vi "Framework Source Test.vi"() -> ()   [LabVIEW 2017]
uses:
  Typedefs/DSF Engine Framework Configuration.ctl
  Typedefs/DSF Engine Plugin Configuration.ctl
  Typedefs/DSF Timing Info.ctl
  Typedefs/DSF Engine Plugin Thread Configuration.ctl
  Typedefs/DSF Settings Info.ctl
  Typedefs/DSF Engine Transfer Group Configuration.ctl
  Typedefs/DSF Direction.ctl
  Typedefs/DSF Engine Transfer Configuration.ctl
  Typedefs/DSF Byte Order.ctl
  Typedefs/DSF Engine Channel Configuration.ctl
  Typedefs/DSF Data Type.ctl
  Typedefs/DSF Timeout Behavior.ctl
  Classes/Framework/Framework Options.ctl
  Typedefs/DSF FIFO Options.ctl
  Classes/Thread/DSF Thread Options.ctl
  Typedefs/DSF Plugin Options.ctl
  Typedefs/DSF Performance Options.ctl
  <vilib>/NI/Memory Manager/Classes/Pointer/Pointer.lvclass/Pointer.ctl
  Classes/Framework/Framework.lvclass/Framework.ctl
  Classes/Performance/Performance.lvclass/Performance.ctl
  Classes/Plugin/Plugin.lvclass/Plugin.ctl
  Classes/Timing/Timing.lvclass/Timing.ctl
  Classes/Transfer Group/Transfer Group.lvclass/Transfer Group.ctl
  Classes/Interface/Interface.lvclass/Interface.ctl
  Classes/Buffers/Buffers.lvclass/Buffers.ctl
  Classes/Framework Status/Framework Status.lvclass/Framework Status.ctl
  <vilib>/NI/Memory Manager/Classes/Pointer/Write Bool.vi
  <vilib>/NI/Memory Manager/Classes/Pointer/Set Address.vi
  <vilib>/NI/Memory Manager/Classes/Pointer/Set Size.vi
  <vilib>/NI/Memory Manager/Classes/Pointer/Set Internal.vi
  <vilib>/NI/Memory Manager/Classes/Pointer/Write (No Check).vi
  <vilib>/NI/Memory Manager/Classes/Pointer/Write (No Check) Bool.vi
  <vilib>/NI/Memory Manager/Classes/Pointer/Check Move.vi
  <vilib>/NI/Memory Manager/Classes/Pointer/Check Null Pointer.vi
  <vilib>/NI/Memory Manager/Classes/Pointer/Clear (No Check).vi
  <vilib>/NI/Memory Manager/Classes/Pointer/Check Length.vi
  <vilib>/NI/Memory Manager/Classes/Pointer/Read (No Check).vi
  <vilib>/NI/Memory Manager/Classes/Pointer/Read (No Check) Bool.vi
  Classes/Framework/Active Plugins.vi
  Classes/Framework/Rx Begin.vi
  Classes/Framework/Rx End.vi
  Classes/Framework/Rx Inline Wait.vi
  Classes/Framework/Rx Async.vi
  Classes/Framework/Rx Inline Start.vi
  Classes/Framework/No Inline Plugins.vi
  Classes/Framework/No Async Plugins.vi
  Classes/Framework/Tx End.vi
  Classes/Framework/Tx Begin.vi
  Classes/Framework/Tx Inline Start.vi
  Classes/Framework/Tx Async.vi
  Classes/Framework/Tx Inline Wait.vi
  Classes/Framework/Update Performance.vi
  Classes/Framework/Update Status.vi
  Classes/Framework/Increment Plugins.vi
  <vilib>/NI/Memory Manager/Classes/Pointer/Get Internal.vi
  <vilib>/NI/Memory Manager/Classes/Pointer/Errors.vi
  <vilib>/NI/Memory Manager/Classes/Pointer/Zone.vi
  <vilib>/NI/Memory Manager/Classes/Pointer/Check Count.vi
  <vilib>/NI/Memory Manager/Classes/Pointer/Check Bounds (Power of 2).vi
  <vilib>/NI/Memory Manager/Classes/Pointer/Null Pointer.vi
  <vilib>/NI/Memory Manager/Classes/Pointer/Is Null.vi
  <vilib>/NI/Memory Manager/Classes/Pointer/Check Bounds (Pointer).vi
  Classes/Plugin/Is Active.vi
  Classes/Plugin/Set Active.vi
  Classes/Plugin/Active Transfer Groups.vi
  Classes/Performance/Rx Begin.vi
  Classes/Performance/Rx End.vi
  Classes/Plugin/Rx Inline Wait.vi
  Classes/Plugin/Rx Async.vi
  Classes/Plugin/Rx Inline Start.vi
  Classes/Performance/Tx End.vi
  Classes/Performance/Tx Begin.vi
  Classes/Plugin/Tx Inline Start.vi
  Classes/Plugin/Tx Async.vi
  Classes/Plugin/Tx Inline Wait.vi
  Classes/Performance/Update Timing.vi
  Classes/Status/Write Status.vi
  Classes/Framework Status/Get Framework Pointer.vi
  Classes/Plugin/Update Status.vi
  Classes/Plugin/Increment Iteration.vi
  <vilib>/NI/Memory Manager/Classes/Pointer/Create Error.vi
  <vilib>/NI/Memory Manager/Classes/Pointer/Out of Bounds.vi
  <vilib>/NI/Memory Manager/Classes/Pointer/Check Bounds.vi
  Classes/Timing/Is Active Cycle.vi
  Classes/Transfer Group/Is Active.vi
  Classes/Transfer Group/Set Active.vi
  Classes/Plugin/Iteration.vi
  Classes/Transfer Group/Wait For Previous.vi
  Classes/Transfer Group/Update Status.vi
  Classes/Transfer Group/Increment Iteration.vi
  Classes/Transfer Group/Get Iteration.vi
  Classes/Thread/Dispatcher/Dispatch Transfer Group.vi
  Classes/Transfer Group/Get ID.vi
  Classes/Transfer Group/Copy Async to Inline.vi
  Classes/Transfer Group/Get Active.vi
  Classes/Plugin/Get ID.vi
  Classes/Transfer Group/Copy Inline to Async.vi
  Classes/Performance/Write Timing Status.vi
  Classes/Status/Status Size.vi
  <vilib>/NI/Memory Manager/Classes/Pointer/Check Size.vi
  Classes/Timing/Get Iteration.vi
  Classes/Timing/Increment Iteration.vi
  <vilib>/NI/Memory Manager/Constants/Constants.vi
  <vilib>/NI/Memory Manager/Constants/Library Name.vi
  <vilib>/NI/Memory Manager/Classes/Pointer/Pointer Error Info.vi
  <vilib>/NI/Memory Manager/Constants/Pointer Class Name.vi
  <vilib>/NI/Memory Manager/Classes/Pointer/Write Pointer Size to Error.vi
  <vilib>/NI/Memory Manager/Classes/Pointer/Check Bounds (Buffer).vi
  Classes/Timing/Get Decimation.vi
  Classes/Timing/Get Offset.vi
  Classes/Plugin/Get Timing.vi
  Classes/Transfer Group/Retrieve from FIFO.vi
  Classes/Interface/Dispatcher/Send Dispatcher Command.vi
  Classes/Buffers/Copy Async to Inline.vi
  Classes/Buffers/Copy Inline to Async.vi
  Classes/Timing Status/Write Timing Status.vi
  <vilib>/NI/Memory Manager/Classes/Pointer/Buffer Underflow.vi
  Classes/Transfer Group/Read Return FIFO.vi
  Classes/Transfer Group/Increment Late Count.vi
  Classes/Interface/Dispatcher/Write Dispatcher Command.vi
  <vilib>/NI/Memory Manager/Classes/Pointer/Copy All.vi
  Classes/Timing Status/Timing Status Size.vi
  Classes/Interface/Send Command.vi
  <vilib>/NI/Memory Manager/Classes/Pointer/Copy.vi
  Classes/Interface/Write RT FIFO.vi
  <vilib>/NI/Memory Manager/Classes/Pointer/Copy (No Check).vi
  Classes/Interface/Dispatcher/Dispatcher Interface.lvclass
  C:/Git/DSF/Core/Classes/Interface/Interface.lvclass
  Classes/Buffer/Buffer.lvclass
  C:/Program Files (x86)/National Instruments/LabVIEW 2017/vi.lib/NI/Memory Manager/Classes/Pointer/Pointer.lvclass
  Classes/Status/Status.lvclass
  Classes/Timing Status/Timing Status.lvclass
  <vilib>/NI/Memory Manager/VIs/New Error Cluster.vi
  <vilib>/NI/Memory Manager/VIs/New Error Cluster (512B).vi
  <vilib>/NI/Memory Manager/VIs/Set Error Status.vi
  <vilib>/NI/Memory Manager/VIs/Set Error Code.vi
  <vilib>/NI/Memory Manager/VIs/Set Error Source.vi
  <vilib>/NI/Memory Manager/VIs/Write String to Source.vi
  <vilib>/NI/Memory Manager/VIs/Write Numeric to Source.vi
  <vilib>/NI/Memory Manager/VIs/Write Numeric Scalar to Source (Base10 U64).vi
  Classes/Interface/Dispatcher/Class Name.vi
  VIs/VI Name.vi
  Classes/Interface/Errors.vi
  Classes/Interface/Dispatcher/Command Timeout.vi
  Classes/Transfer Group/Errors.vi
  Classes/Transfer Group/Invalid Iteration Error.vi
  Classes/Transfer Group/Return Timeout Error.vi
  <vilib>/NI/Memory Manager/Classes/Pointer/Pointer.lvclass
  Classes/Framework/Framework.lvclass
  <vilib>/NI/Memory Manager/Classes/Pointer/Read Bool.vi
  Classes/Configuration/Configuration Session.lvclass
  DSF Core.lvlib
panel:
  in  "components directory":path
  in  "dsf configuration file path":path=path "C:/Users/Admin/Desktop/test.dsf"
  out "iteration":u64
  out "error out":errorcluster
  in  "framework options":T1={"FIFO Options"={"Infinite Timeouts"=TRUE}, "Thread Options"={"Show FP On Call"=TRUE, "Close FP After Call"=TRUE, "Allow Debugging"=TRUE}, "Plugin Options"={"Default Components"=TRUE}, "Performance Options"={"Measure Period"=TRUE, "Measure Rx/Tx Duration"=TRUE}}
  in  "framework configuration":T6={"Plugins"=[{"name"="UDP", "components"=["UDP"], "cycle timing"={"priority"=100, "decimation"=1, "offset"=0}, "threads"=[{"buffer converter settings"=[], "transceiver settings"=[{"key"="Local Port", "value"="50000"}], "custom settings"=[], "processor"=-2, "priority offset"=0}, {"buffer converter settings"=[], "transceiver settings"=[{"key"="Local Port", "value"="50001"}], "custom settings"=[], "processor"=-2, "priority offset"=0}, {"buffer converter settings"=[], "transceiver settings"=[{"key"="Local Port", "value"="50002"}], "custom settings"=[], "processor"=-2, "priority offset"=0}, {"buffer converter settings"=[], "transceiver settings"=[{"key"="Local Port", "value"="50003"}], "custom settings"=[], "processor"=-2, "priority offset"=0}], "Transfer Groups"=[{"name"="Group0", "direction"=enum."Tx", "cycle timing"={"priority"=100, "decimation"=1, "offset"=0}, "thread index"=0, "settings"=[], "Transfers"=[{"name"="Transfer0", "byte order"=enum."big-endian", "settings"=[{"key"="Destination Port", "value"="60000"}, {"key"="Destination Address", "value"="localhost"}], "channels"=[{"string offset"=0, "string data type"=enum."SGL", "engine data type"=enum."DBL", "name"="Temp", "settings"=[], "units"="V"}, {"string offset"=4, "string data type"=enum."DBL", "engine data type"=enum."DBL", "name"="RPM", "settings"=[], "units"="V"}, {"string offset"=12, "string data type"=enum."Bool", "engine data type"=enum."DBL", "name"="LED", "settings"=[], "units"="V"}, {"string offset"=792, "string data type"=enum."U64", "engine data type"=enum."DBL", "name"="Count", "settings"=[], "units"="V"}]}], "timeout behavior"=enum."Increment Late Count"}], "settings"=[]}]}
  in  "stop":bool
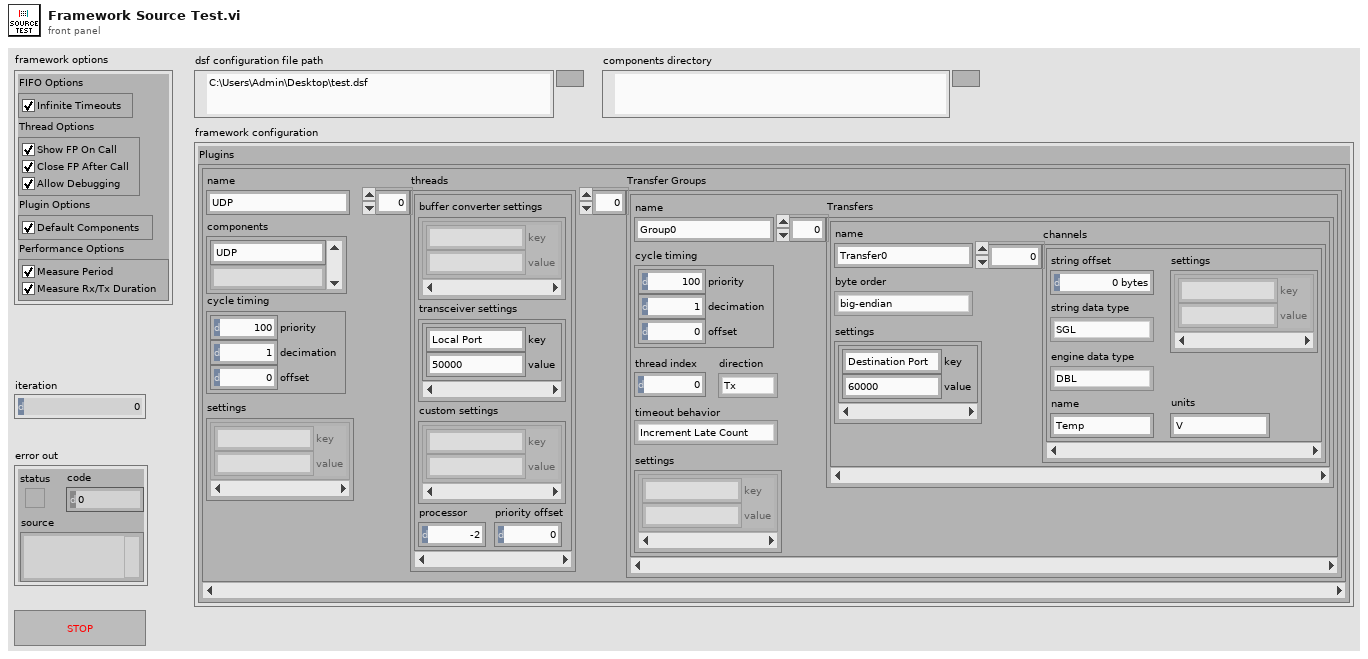
[diagram p1: front panel]
types:
  T1 = typedef "DSF Core.lvlib/Framework.lvclass/Framework Options.ctl" = cluster{"FIFO Options":T2, "Thread Options":T3, "Plugin Options":T4, "Performance Options":T5}
  T2 = typedef "DSF Core.lvlib/DSF FIFO Options.ctl" = cluster{"Infinite Timeouts":bool}
  T3 = typedef "DSF Core.lvlib/DSF Thread Options.ctl" = cluster{"Show FP On Call":bool, "Close FP After Call":bool, "Allow Debugging":bool}
  T4 = typedef "DSF Core.lvlib/DSF Plugin Options.ctl" = cluster{"Default Components":bool}
  T5 = typedef "DSF Core.lvlib/DSF Performance Options.ctl" = cluster{"Measure Period":bool, "Measure Rx/Tx Duration":bool}
  T6 = typedef "DSF Core.lvlib/DSF Engine Framework Configuration.ctl" = cluster{"Plugins":T7[]}
  T7 = typedef "DSF Core.lvlib/DSF Engine Plugin Configuration.ctl" = cluster{"name":string, "components":string[], "cycle timing":T8, "threads":T9[], "Transfer Groups":T11[], "settings":T10}
  T8 = typedef "DSF Core.lvlib/DSF Timing Info.ctl" = cluster{"priority":u64, "decimation":u64, "offset":u64}
  T9 = typedef "DSF Core.lvlib/DSF Engine Plugin Thread Configuration.ctl" = cluster{"buffer converter settings":T10, "transceiver settings":T10, "custom settings":T10, "processor":i32, "priority offset":i16}
  T10 = typedef "DSF Core.lvlib/DSF Settings Info.ctl" = cluster{"key":string, "value":string}[]
  T11 = typedef "DSF Core.lvlib/DSF Engine Transfer Group Configuration.ctl" = cluster{"name":string, "direction":T12, "cycle timing":T8, "thread index":i32, "settings":T10, "Transfers":T13[], "timeout behavior":T17}
  T12 = typedef "DSF Core.lvlib/DSF Direction.ctl" = enum8{"Tx", "Rx"}
  T13 = typedef "DSF Core.lvlib/DSF Engine Transfer Configuration.ctl" = cluster{"name":string, "byte order":T14, "settings":T10, "channels":T15[]}
  T14 = typedef "DSF Core.lvlib/DSF Byte Order.ctl" = enum8{"big-endian", "little-endian"}
  T15 = typedef "DSF Core.lvlib/DSF Engine Channel Configuration.ctl" = cluster{"string offset":u64, "string data type":T16, "engine data type":T16, "name":string, "settings":T10, "units":string}
  T16 = typedef "DSF Core.lvlib/DSF Data Type.ctl" = enum8{"Bool", "SGL", "DBL", "I8", "I16", "I32", "I64", "U8", "U16", "U32", "U64"}
  T17 = typedef "DSF Core.lvlib/DSF Timeout Behavior.ctl" = enum8{"Increment Late Count", "Throw Error"}
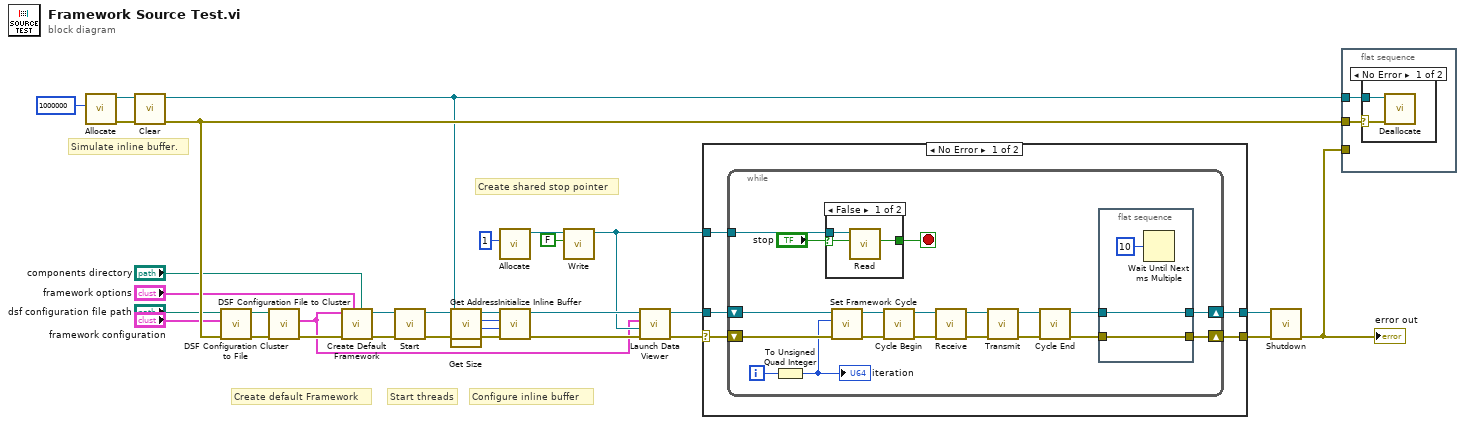
[diagram p0: block diagram]
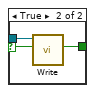
[diagram p3: hidden frame]
diagram:
  # "Create shared stop pointer"
  # "Configure inline buffer"
  # "Start threads"
  # "Create default Framework"
  # "Simulate inline buffer."
  n1 = call <vilib>:"Allocate.vi"("size"=u64 1000000) -> ("error out"=w24:errorcluster, "Pointer out"=w17:refnum<class "Pointer.lvclass">)  [unwired: 9 in]
  n2 = call <vilib>:"Clear.vi"("error in (no error)"=w24, "Pointer in"=w17) -> ("error out"=w29:errorcluster, "Pointer out"=w2:refnum<class "Pointer.lvclass">)  [unwired: 8 in]
  n3 = call "DSF Configuration Cluster to File.vi"("error in (no error)"=w29, "framework configuration"="framework configuration", "dsf configuration file path"="dsf configuration file path") -> ("error out"=w23:errorcluster, "dsf configuration file path dup"=w22:path)  [unwired: 7 in]
  n4 = call "DSF Configuration File to Cluster.vi"("error in (no error)"=w23, "dsf configuration file path"=w22) -> ("error out"=w16:errorcluster, "framework configuration out"=w4:T6)  [unwired: 7 in, 1 out]
  n5 = call "Create Default Framework.vi"("components directory (default)"="components directory", "framework options"="framework options", "error in (no error)"=w16, "framework configuration"=w4) -> ("error out"=w1:errorcluster, "Framework"=w13:refnum<class "Framework.lvclass">)  [unwired: 6 in]
  n6 = call-dynamic "Start.vi"("error in (no error)"=w1, "Framework in"=w13) -> ("error out"=w12:errorcluster, "Framework out"=w30:refnum<class "Framework.lvclass">)  [unwired: 8 in]
  n7 = call <vilib>:"Get Address.vi"("Pointer in"=w2) -> ("address"=w20:u64)  [unwired: 9 in, 1 out]
  n8 = call <vilib>:"Get Size.vi"("Pointer in"=w2) -> ("size"=w21:u64)  [unwired: 9 in, 1 out]
  n9 = call <vilib>:"Allocate.vi"("size"=u64 1) -> ("Pointer out"=w8:refnum<class "Pointer.lvclass">)  [unwired: 9 in, 1 out]
  n10 = call "Initialize Inline Buffer.vi"("error in (no error)"=w12, "size"=w21, "address"=w20, "Framework in"=w30) -> ("error out"=w10:errorcluster, "Framework out"=w11:refnum<class "Framework.lvclass">)  [unwired: 6 in]
  n11 = call-poly <vilib>:"Write.vi"("value"=FALSE, "Pointer in"=w8) -> ("Pointer out"=w7:refnum<class "Pointer.lvclass">)  [unwired: 6 in, 3 out]
  n12 = call "Launch Data Viewer.vi"("error in (no error)"=w10, "Stop Pointer"=w7, "Framework Configuration"=w4, "Framework in"=w11) -> ("error out"=w18:errorcluster, "Framework out"=w19:refnum<class "Framework.lvclass">)  [unwired: 6 in]
  n13 = case shown="No Error" w18 {
    selector: w18 -> [w34 w64]
    tunnel: [w32 w64] -> w28
    tunnel: w19 -> [w35 w65]
    tunnel: [w33 w65] -> w27
    tunnel: w7 -> [w31 _]
    frame No Error {
      n14 = while {
        shift-right: [w52] -> w33
        shift-left: w35 -> [w44]
        shift-right: [w51] -> w32
        shift-left: w34 -> [w43]
        tunnel: w31 -> [w49]
        i -> [w50]
        stop <- w47 stop-if-true
        n15 = To Unsigned Quad Integer(1:w50) -> (0:w42:u64)
        "iteration" <- w42
        n16 = case shown="False" "stop" {
          selector: "stop" -> [w56 w59]
          tunnel: w49 -> [w57 w60]
          tunnel: [w55 w58] -> w47
          frame False {
            n17 = call-poly <vilib>:"Read.vi"("value in"=w56, "Pointer in"=w57) -> ("value out"=w55:bool)  [unwired: 6 in, 3 out]
          }
          frame True {
            n18 = call-poly <vilib>:"Write.vi"("value"=w59, "Pointer in"=w60) -> ("value"=w58:bool)  [unwired: 6 in, 3 out]
          }
        }
        n19 = call "Set Framework Cycle.vi"("error in (no error)"=w43, "iteration"=w42, "Framework in"=w44) -> ("error out"=w40:errorcluster, "Framework out"=w41:refnum<class "Framework.lvclass">)  [unwired: 7 in]
        n20 = call "Cycle Begin.vi"("error in (no error)"=w40, "Framework in"=w41) -> ("error out"=w38:errorcluster, "Framework out"=w39:refnum<class "Framework.lvclass">)  [unwired: 8 in]
        n21 = call "Receive.vi"("error in (no error)"=w38, "Framework in"=w39) -> ("error out"=w54:errorcluster, "Framework out"=w53:refnum<class "Framework.lvclass">)  [unwired: 8 in]
        n22 = call "Transmit.vi"("error in (no error)"=w54, "Framework in"=w53) -> ("error out"=w36:errorcluster, "Framework out"=w37:refnum<class "Framework.lvclass">)  [unwired: 8 in]
        n23 = call "Cycle End.vi"("error in (no error)"=w36, "Framework in"=w37) -> ("error out"=w45:errorcluster, "Framework out"=w46:refnum<class "Framework.lvclass">)  [unwired: 8 in]
        n24 = flat-sequence {
          tunnel: w46 -> [w62]
          tunnel: w45 -> [w61]
          tunnel: [w62] -> w52
          tunnel: [w61] -> w51
          frame #0 {
            n25 = Wait Until Next ms Multiple(millisecond multiple=u32 10 ("milliseconds to wait")) -> ()  [unwired: 1 out]
          }
        }
      }
    }
    frame Error {
    }
  }
  n26 = call-dynamic "Shutdown.vi"("error in (no error)"=w28, "Framework in"=w27) -> ("error out"=w25:errorcluster)  [unwired: 8 in, 1 out]
  "error out" <- w25
  n27 = flat-sequence {
    tunnel: w2 -> [w67]
    tunnel: w25 -> [_]
    tunnel: w29 -> [w66]
    frame #0 {
      n28 = case shown="No Error" w66 {
        selector: w66 -> [w68 _]
        tunnel: w67 -> [w69 _]
        frame No Error {
          n29 = call <vilib>:"Deallocate.vi"("error in (no error)"=w68, "Pointer"=w69) -> ()  [unwired: 8 in, 2 out]
        }
        frame Error {
        }
      }
    }
  }
